vi "RealBLDC_Acquisition.vi"() -> ()   [LabVIEW 2018]
doc: "VI criada para realizar a aquisição de sinais do motor real e salvá-los em arquivo."
uses:
  controls/RealBLDC - States.ctl
  controls/RealBLDC - Data.ctl
  <vilib>/DAQmx/read.llb/DAQmx Read (Analog DBL 1Chan 1Samp).vi
  <vilib>/DAQmx/create/channels.llb/DAQmx Create Channel (AI-Voltage-Basic).vi
  <vilib>/DAQmx/create/channels.llb/DAQmx Create Channel (AI-Current-Basic).vi
  <vilib>/DAQmx/miscellaneous.llb/DAQmx Fill In Error Info.vi
panel:
  in  "Leitura de Corrente":tag
  in  "Leitura de Tensão":tag
  in  "Teste Corrente":path
  in  "Teste Tensão":path
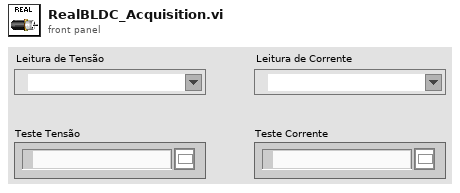
[diagram p1: front panel]
types:
  T1 = typedef "RealBLDC - Data.ctl" = cluster{"Tensão task":refnum<k21>, "Corrente task":refnum<k21>, "Teste Tensão ":refnum<k34>, "Teste Corrente":refnum<k34>}
  T2 = typedef "RealBLDC - States.ctl" = enum16{"Initialize", "Acquire", "Exit"}
  T3 = enum16{"open", "open or create", "create or replace", "create", "open (read-only)"}
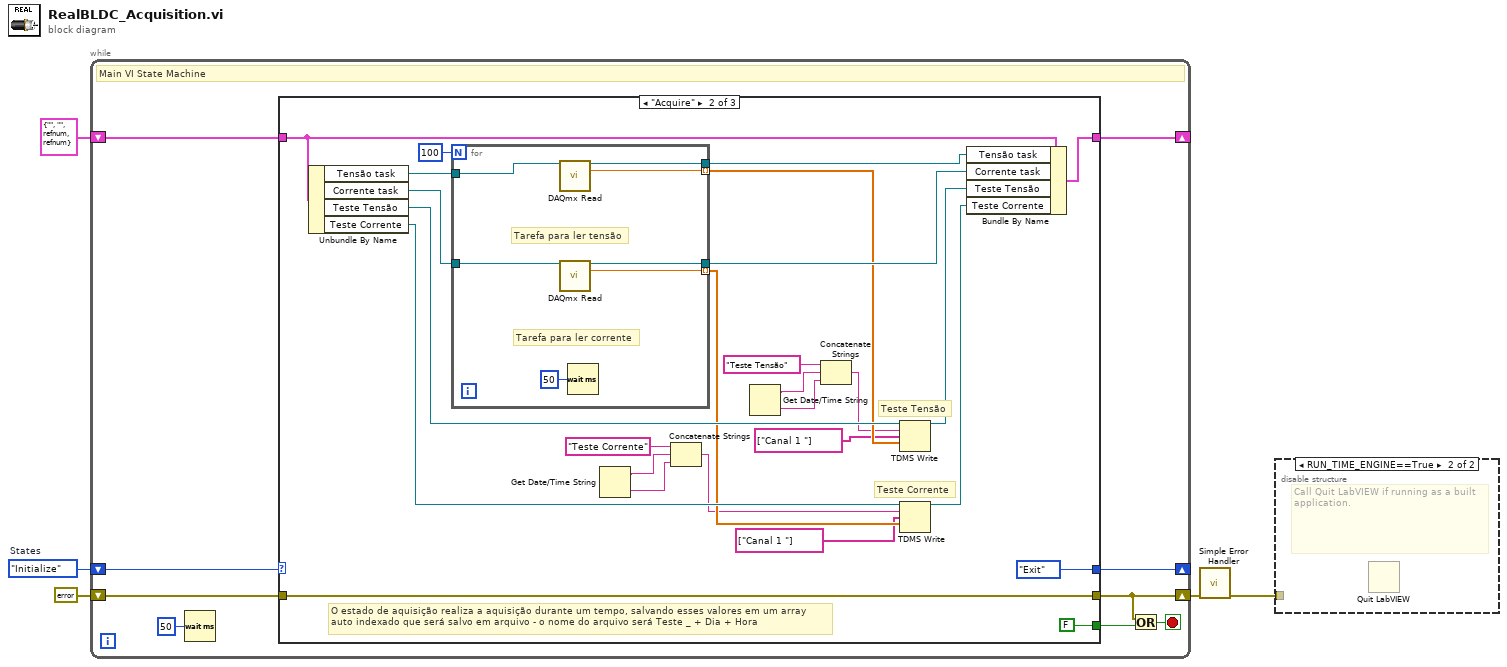
[diagram p0: block diagram]
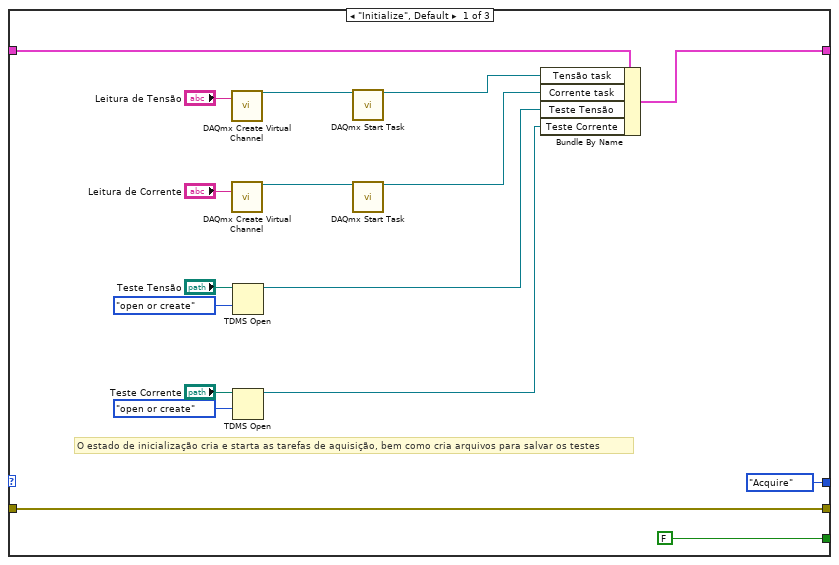
[diagram p3: hidden frame]
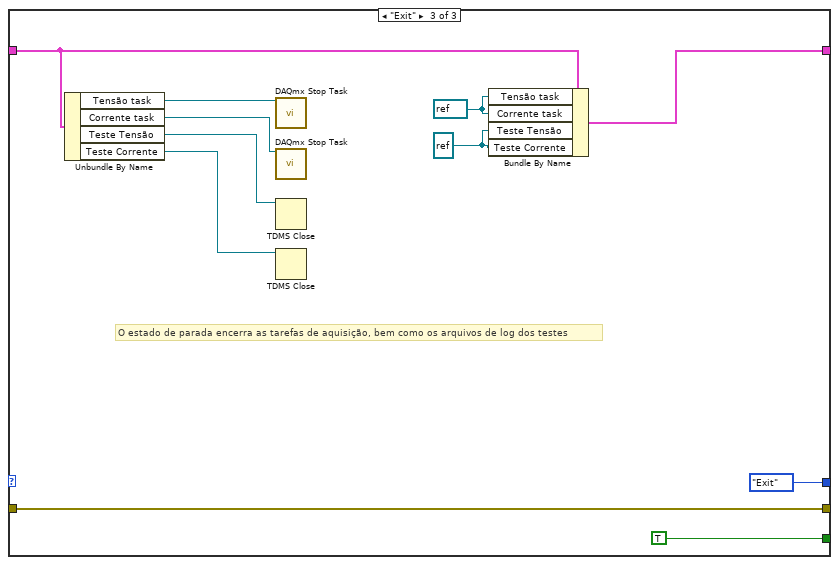
[diagram p4: hidden frame]
diagram:
  w1 = RealBLDC_-_States."Initialize"  # States
  n1 = while {
    shift-right: [w8] -> _
    shift-left: w1 -> [w6]
    shift-right: [w10] -> w4
    shift-left: errorcluster {"status"=FALSE, "code"=0, "source"=""} ("error constant") -> [w11]
    shift-right: [w12] -> _
    shift-left: T1 {"Tensão task"="", "Corrente task"="", "Teste Tensão "=refnum, "Teste Corrente"=refnum} -> [w13]
    stop <- w14 stop-if-true
    # "Main VI State Machine"
    n2 = Wait (ms)(milliseconds to wait=u32 50) -> ()  [unwired: 1 out]
    n3 = case shown="\"Acquire\"" w6 {
      tunnel: w13 -> [w25 w51 w68]
      tunnel: [w24 w50 w67] -> w12
      tunnel: w11 -> [w19 w57 w75]
      tunnel: [w19 w57 w75] -> w10
      tunnel: [FALSE FALSE TRUE] -> w9
      tunnel: [RealBLDC_-_States."Acquire" ("Next State") RealBLDC_-_States."Exit" ("Next State") RealBLDC_-_States."Exit" ("Next State")] -> w8
      frame "Initialize", Default {
        # "O estado de inicialização cria e starta as tarefas de aquisição, bem como cria arquivos para salvar os testes"
        n4 = call-poly <vilib>:"DAQmx Create Virtual Channel.vi"("physical channels"="Leitura de Tensão") -> ("task out"=w31:refnum<k21>)  [unwired: 13 in, 1 out]
        n5 = call-poly <vilib>:"DAQmx Create Virtual Channel.vi"("physical channels"="Leitura de Corrente") -> ("task out"=w28:refnum<k21>)  [unwired: 13 in, 1 out]
        n6 = TDMS Open(10:T3."open or create" ("operation (0:open)"), 11:"Teste Tensão") -> (3:w21:refnum<k34>)  [unwired: 5 in, 1 out]
        n7 = TDMS Open(10:T3."open or create" ("operation (0:open)"), 11:"Teste Corrente") -> (3:w22:refnum<k34>)  [unwired: 5 in, 1 out]
        n8 = call <vilib>:"DAQmx Start Task.vi"("task/channels in"=w31) -> ("task out"=w23:refnum<k21>)  [unwired: 13 in, 1 out]
        n9 = call <vilib>:"DAQmx Start Task.vi"("task/channels in"=w28) -> ("task out"=w20:refnum<k21>)  [unwired: 13 in, 1 out]
        n10 = Bundle By Name(cluster=w25, "Tensão task"=w23, "Corrente task"=w20, "Teste Tensão"=w21, "Teste Corrente"=w22) -> (w24:T1)
      }
      frame "Acquire" {
        # "O estado de aquisição realiza a aquisição durante um tempo, salvando esses valores em um array auto indexado que será salvo em arquivo - o nome do arquivo será Teste _ + Dia + Hora"
        # "Teste Corrente"
        # "Teste Tensão"
        n11 = Unbundle By Name(w51) -> ("Tensão task"=w53:refnum<k21>, "Corrente task"=w52:refnum<k21>, "Teste Tensão"=w47:refnum<k34>, "Teste Corrente"=w46:refnum<k34>)
        n12 = for {
          N: 100 -> [_]
          tunnel: w53 -> [w64]
          tunnel: w52 -> [w63]
          tunnel: [w62] -> w43 mode=indexing
          tunnel: [w61] -> w49
          tunnel: [w60] -> w42 mode=indexing
          tunnel: [w59] -> w48
          # "Tarefa para ler corrente"
          # "Tarefa para ler tensão"
          n13 = call-poly <vilib>:"DAQmx Read.vi"("task/channels in"=w64) -> ("task out"=w61:refnum<k21>, "data"=w62:dbl)  [unwired: 12 in, 1 out]
          n14 = call-poly <vilib>:"DAQmx Read.vi"("task/channels in"=w63) -> ("task out"=w59:refnum<k21>, "data"=w60:dbl)  [unwired: 12 in, 1 out]
          n15 = Wait (ms)(milliseconds to wait=u32 50) -> ()  [unwired: 1 out]
        }
        n16 = Get Date/Time String() -> (date string=w34:string, time string=w35:string)  [unwired: 3 in]
        n17 = Concatenate Strings("Teste Corrente" ("string"), w34, w35) -> (w32:string)
        n18 = Get Date/Time String() -> (date string=w40:string, time string=w39:string)  [unwired: 3 in]
        n19 = Concatenate Strings("Teste Tensão" ("string"), w40, w39) -> (w38:string)
        n20 = TDMS Write(0:w47, 5:w38, 7:string[] ["Canal 1 "] ("channel name(s) in (Untitled)"), 9:w43) -> (4:w45:refnum<k34>)  [unwired: 2 in, 3 out]
        n21 = TDMS Write(0:w46, 5:w32, 7:string[] ["Canal 1 "] ("channel name(s) in (Untitled)"), 9:w42) -> (4:w44:refnum<k34>)  [unwired: 2 in, 3 out]
        n22 = Bundle By Name(cluster=w51, "Tensão task"=w49, "Corrente task"=w48, "Teste Tensão"=w45, "Teste Corrente"=w44) -> (w50:T1)
      }
      frame "Exit" {
        w66 = refnum<k21> refnum ("task out")
        w65 = refnum<k34> refnum ("tdms file out")
        # "O estado de parada encerra as tarefas de aquisição, bem como os arquivos de log dos testes"
        n23 = Unbundle By Name(w68) -> ("Tensão task"=w72:refnum<k21>, "Corrente task"=w71:refnum<k21>, "Teste Tensão"=w70:refnum<k34>, "Teste Corrente"=w69:refnum<k34>)
        n24 = call <vilib>:"DAQmx Stop Task.vi"("task/channels in"=w72) -> ()  [unwired: 13 in, 2 out]
        n25 = call <vilib>:"DAQmx Stop Task.vi"("task/channels in"=w71) -> ()  [unwired: 13 in, 2 out]
        n26 = TDMS Close(11:w70) -> ()  [unwired: 1 in, 2 out]
        n27 = TDMS Close(11:w69) -> ()  [unwired: 1 in, 2 out]
        n28 = Bundle By Name(cluster=w68, "Tensão task"=w66, "Corrente task"=w66, "Teste Tensão"=w65, "Teste Corrente"=w65) -> (w67:T1)
      }
    }
    n29 = Or(x=w10, y=w9) -> (x .or. y?=w14:bool)
  }
  n30 = call <vilib>:"Simple Error Handler.vi"("error in (no error)"=w4) -> ("error out"=w3:errorcluster)  [unwired: 4 in, 4 out]
  n31 = disable-structure shown="RUN_TIME_ENGINE==True" {
    disable-tunnel: w3 -> [_ _]
    frame condition #0 (active) {
    }
    frame condition #1 {
      # "Call Quit LabVIEW if running as a built application."
      n32 = Quit LabVIEW() -> ()  [unwired: 1 in]
    }
  }
